vi "Digital Input DAQ Setup.vi"(4 "samples per channel":i32=1000, 6 "rate":dbl=1000.0 format="%0.2f", 8 "error in":errorcluster, 9 "name to assign":string, 10 "Condensate Flow Rate Channel":tag, 11 "task/channels in":refnum<k21>) -> (0 "error out":errorcluster, 3 "Refnum out":refnum<k21>)   [LabVIEW 2017]
uses:
  <vilib>/DAQmx/create/channels.llb/DAQmx Create Channel (DI-Digital Input).vi
  <vilib>/DAQmx/configure/timing.llb/DAQmx Timing (Sample Clock).vi
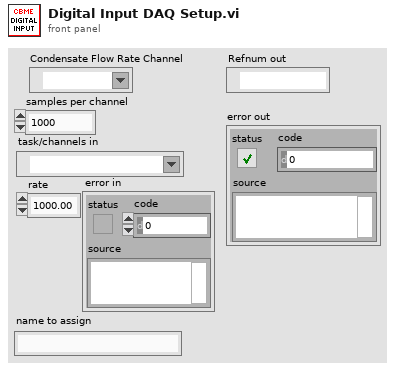
[diagram p1: front panel]
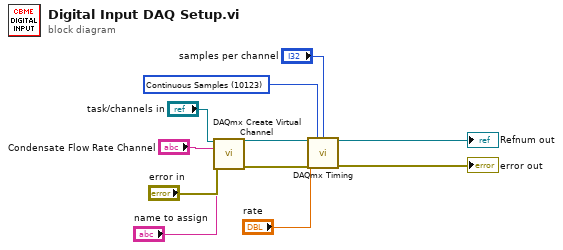
[diagram p0: block diagram]
diagram:
  w2 = 10123 items=["Finite Samples"=10178, "Continuous Samples"=10123, "Hardware Timed Single Point"=12522] ("sample mode")
  n1 = call-poly <vilib>:"DAQmx Create Virtual Channel.vi"("task in"="task/channels in", "lines"="Condensate Flow Rate Channel", "name to assign"="name to assign", "error in"="error in") -> ("task out"=w8:refnum<k21>, "error out"=w9:errorcluster)  [unwired: 10 in]
  n2 = call-poly <vilib>:"DAQmx Timing.vi"("task/channels in"=w8, "sample mode"=w2, "samples per channel"="samples per channel", "rate"="rate", "error in"=w9) -> ("task out"=→"Refnum out":refnum<k21>, "error out"=→"error out":errorcluster)  [unwired: 9 in]
